vi "Send Details to Container.vi"(8 "error in (no error)":errorcluster, 11 "GUI View Actor in":refnum<class "GUI View Actor.lvclass">) -> (0 "error out":errorcluster, 3 "GUI View Actor out":refnum<class "GUI View Actor.lvclass">)   [LabVIEW 2017, in "GUI Views.lvlib" / "GUI View Actor.lvclass"]
uses:
  GUI View Actor.lvclass
  C:/Program Files/National Instruments/LabVIEW 2017/vi.lib/ActorFramework/Actor/Actor.lvclass
  C:/Projects/Shared Libraries/Event Actors/View Actor/View Actor.lvclass
  GUI View Actor.lvclass/GUI View Actor.ctl
  GUI Container Actor/typedefs/View Details.ctl
  <vilib>/ActorFramework/Message Enqueuer/Message Enqueuer.lvclass
  <vilib>/ActorFramework/Actor/Actor.lvclass/Actor.ctl
  <vilib>/ActorFramework/Message Enqueuer/Message Enqueuer.lvclass/Message Enqueuer.ctl
  View Actor/View Actor.lvclass/View Actor.ctl
  View Actor/properties/Read Name.vi
  properties/Read Managed by Container.vi
  <vilib>/ActorFramework/Message Enqueuer/Init from Existing Queue.vi
  <vilib>/ActorFramework/Message Enqueuer/Equals Not A Refnum.vi
  GUI Container Actor Messages/Add View Msg/Add View Msg.lvclass
  GUI Container Actor/GUI Container Actor.lvclass
  <vilib>/ActorFramework/Actor/Actor.lvclass
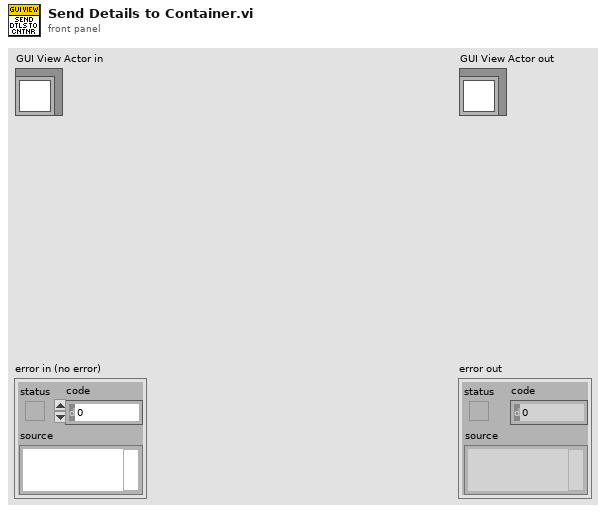
[diagram p1: front panel]
types:
  T1 = typedef "GUI Views.lvlib/GUI Container Actor.lvclass/View Details.ctl" = cluster{"Enqueuer":refnum<class "Message Enqueuer.lvclass">, "VI References":refnum<vi>[], "FP References":refnum<vi>[]}
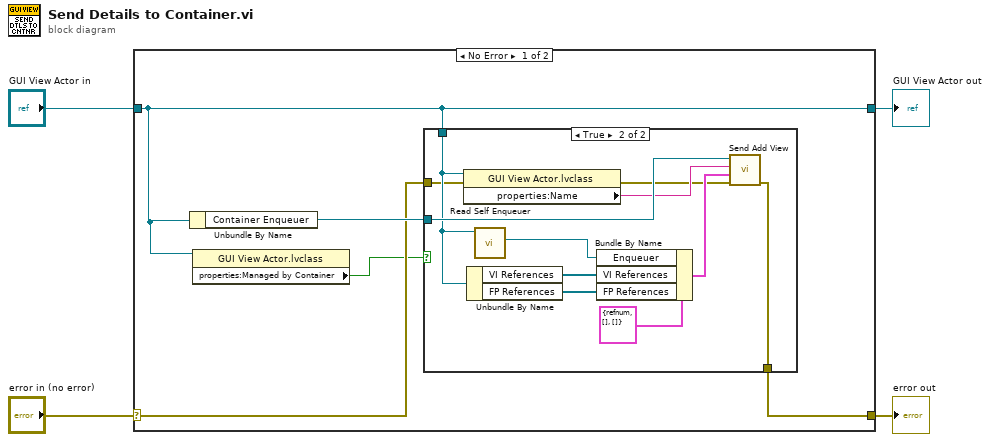
[diagram p0: block diagram]
diagram:
  n1 = case shown="No Error" "error in (no error)" {
    selector: "error in (no error)" -> [w8 w23]
    tunnel: [w7 w23] -> w3
    tunnel: [w6 w22] -> w1
    tunnel: "GUI View Actor in" -> [w6 w22]
    frame No Error {
      n2 = Unbundle By Name(w6) -> ("Container Enqueuer"=w9:refnum<class "Message Enqueuer.lvclass">)
      n3 = property class="GUI View Actor.lvclass"(reference=w6) -> ("properties:Managed by Container"=w5:bool)  [unwired: 1 in, 2 out]
      n4 = case shown="True" w5 {
        tunnel: w9 -> [_ w21]
        tunnel: w6 -> [_ w17]
        tunnel: w8 -> [w10 w13]
        tunnel: [w10 w12] -> w7
        frame False {
        }
        frame True {
          n5 = property class="GUI View Actor.lvclass"(reference=w17, error in=w13) -> (error out=w14:errorcluster, "properties:Name"=w20:string)  [unwired: 1 out]
          n6 = Unbundle By Name(w17) -> ("VI References"=w11:refnum<vi>[], "FP References"=w18:refnum<vi>[])
          n7 = call <vilib>:"Read Self Enqueuer.vi"("Actor"=w17) -> ("Self Enqueuer"=w16:refnum<class "Message Enqueuer.lvclass">)  [unwired: 10 in]
          n8 = Bundle By Name(cluster=T1 {"Enqueuer"=refnum, "VI References"=[], "FP References"=[]} ("View Details"), "Enqueuer"=w16, "VI References"=w11, "FP References"=w18) -> (w15:T1)
          n9 = call "Send Add View.vi"("error in (no error)"=w14, "View Details"=w15, "View"=w20, "Message Enqueuer in"=w21) -> ("error out"=w12:errorcluster)  [unwired: 6 in, 1 out]
        }
      }
    }
    frame Error {
    }
  }
  "error out" <- w3
  "GUI View Actor out" <- w1
